vi "Find script.vi"(8 "error in (no error)":errorcluster, 10 "Script name":string, 11 "FPGA Interface":refnum<class "FPGA Interface.lvclass">) -> (0 "error out":errorcluster, 2 "Found?":bool, 3 "Script path":path)   [LabVIEW 2026, in "TALOS.lvlib" / "Interfaces.lvlib" / "FPGA Interface.lvclass"]
doc: "Vi for finding paths of scripts updated directly from the GUI. The entry is updated if the path is found. Otherwise the entry is deleted from the array. It looks for the scripts in th <ARTIQ_Codes>\\Scripts path and ignores Archive folders."
uses:
  FPGA Interface.lvclass
panel:
  # "For debug only"
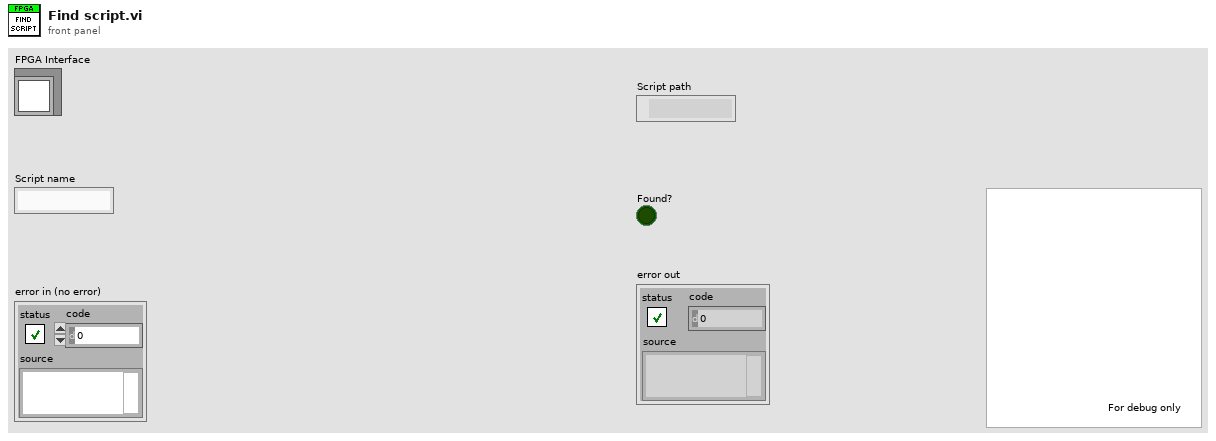
[diagram p1: front panel]
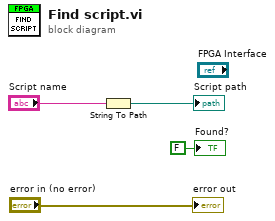
[diagram p0: block diagram]
diagram:
  n1 = String To Path(string="Script name") -> (path=→"Script path":path)
  "error out" <- "error in (no error)"
  "Found?" <- FALSE ("Found?")
